vi "getWaveform daq.vi"(1 "df":dbl[](array[numeric]), 2 "Fs (S/s)":dbl, 3 "#samples":u32) -> (0 "Waveform":waveform(dbl)(graph))   [LabVIEW 2010]
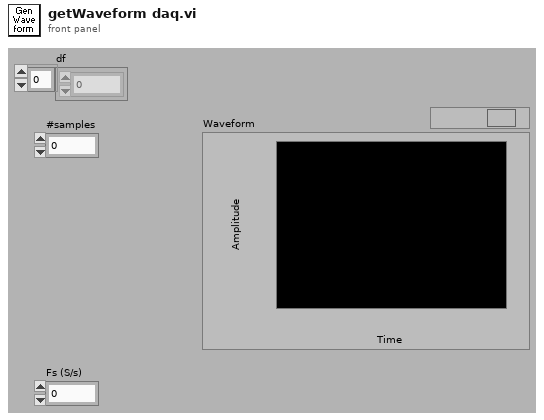
[diagram p1: front panel]
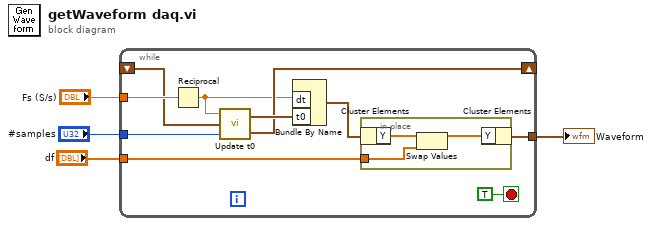
[diagram p0: block diagram]
diagram:
  n1 = while {
    tunnel: "#samples" -> [w8]
    tunnel: "Fs (S/s)" -> [w13]
    shift-right: [w9] -> _
    shift-left: _ -> [w11]
    tunnel: [w6] -> w4
    tunnel: "df" -> [w5]
    stop <- TRUE stop-if-true
    n2 = Reciprocal(x=w13) -> (1/x=w7:dbl)
    n3 = call "Update t0.vi"("#samples"=w8, "t0 IN"=w11, "dt"=w7) -> ("tf new"=w9:timestamp, "t0 OUT"=w10:timestamp)
    n4 = Bundle By Name("dt"=w7, "t0"=w10) -> (w12:waveform(dbl))  [unwired: 1 in]
    n5 = in-place {
      in-place-border: w5 -> [w15]
      n6 = in-place-cluster #1(w12) -> ("Y"=w17:dbl[])
      n7 = Swap Values(12:w17, 14:w15) -> (1:w16:dbl[])  [unwired: 1 in, 1 out]
      n8 = in-place-cluster #1("Y"=w16) -> (w6:waveform(dbl))
    }
  }
  "Waveform" <- w4
